vi "to_U8.vi"(8 "error_in":errorcluster, 10 "variable_start_index":i32, 11 "byte_array":u8[](array[numeric])) -> (0 "error_out":errorcluster, 3 "U8":u8)   [LabVIEW 2020]
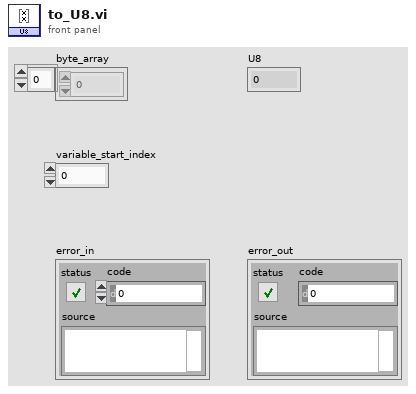
[diagram p1: front panel]
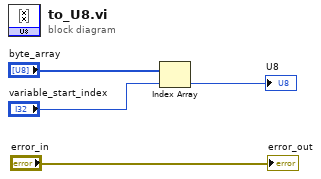
[diagram p0: block diagram]
diagram:
  n1 = Index Array(array="byte_array", index="variable_start_index") -> (element=→"U8":u8)
  "error_out" <- "error_in"
